vi "Read Service.vi"(8 "error in (no error)":errorcluster, 11 "AWS Core in":refnum<class "AWS Core.lvclass">) -> (0 "error out":errorcluster, 2 "Service":string, 3 "AWS Core out":refnum<class "AWS Core.lvclass">)   [LabVIEW 2015, in "NI_AWS Core.lvlib" / "AWS Core.lvclass"]
uses:
  AWS Core.lvclass
  AWS Core.lvclass/AWS Core.ctl
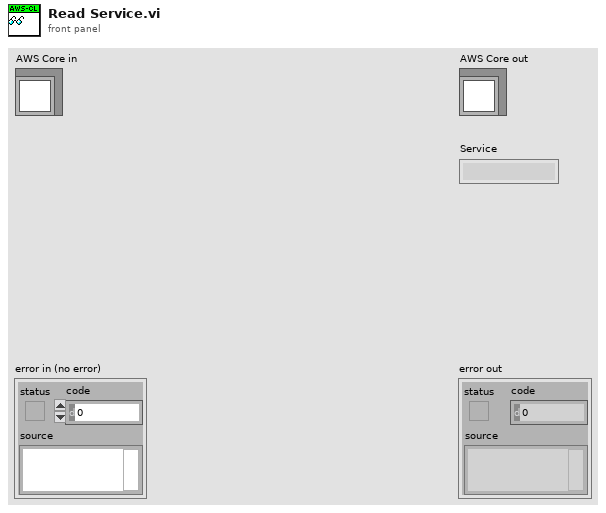
[diagram p1: front panel]
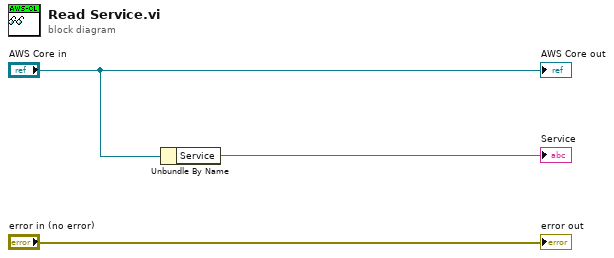
[diagram p0: block diagram]
diagram:
  n1 = Unbundle By Name("AWS Core in") -> ("Service"=→"Service":string)
  "error out" <- "error in (no error)"
  "AWS Core out" <- "AWS Core in"
